vi "Write to RAM.vi"(8 "error in (no error)":errorcluster, 9 "data":u8[](array[numeric]), 10 "address":u16, 11 "TroSpec in":refnum<class "PL ISTEQ TroSpec.lvclass">) -> (0 "error out":errorcluster, 3 "TroSpec out":refnum<class "PL ISTEQ TroSpec.lvclass">)   [LabVIEW 2015, in "PL ISTEQ TroSpec.lvclass"]
doc: "Writes data to RAM."
uses:
  PL ISTEQ TroSpec.lvclass
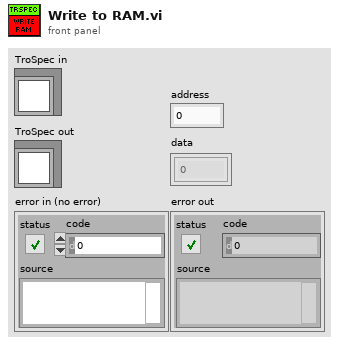
[diagram p1: front panel]
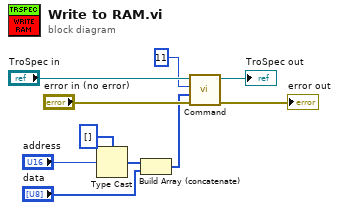
[diagram p0: block diagram]
diagram:
  n1 = Type Cast(type=u8[] [] ("command payload"), x="address") -> (*(type *) &x=w3:u8[])
  n2 = Build Array (concatenate)(w3, "data") -> (w2:u8[])
  n3 = call "Command.vi"("error in (no error)"="error in (no error)", "command payload"=w2, "command"=u8 11, "TroSpec in"="TroSpec in") -> ("error out"=→"error out":errorcluster, "TroSpec out"=→"TroSpec out":refnum<class "PL ISTEQ TroSpec.lvclass">)  [unwired: 5 in, 1 out]
